vi "Send Create Arbitrary Sequence [SEQ].vi"(7 "Message Priority (Normal)":T1=enum."Normal", 8 "error in (no error)":errorcluster, 9 "waveform handles array (empty)":i32[](array[numeric]), 10 "loop counts array (empty)":i32[](array[numeric]), 11 "Message Enqueuer":refnum<class "Message Enqueuer.lvclass">) -> (0 "error out":errorcluster, 3 "Message Enqueuer out":refnum<class "Message Enqueuer.lvclass">)   [LabVIEW 2015, in "CS++Fgen.lvlib" / "Create Arbitrary Sequence [SEQ] Msg.lvclass"]
doc: "Sends the <B>CS++Fgen.lvlib:Create Arbitrary Sequence [SEQ] Msg.lvclass</B> message.\n\n<B>CS++Fgen.lvlib:CS++Fgen.lvclass:Create Arbitrary Sequence [SEQ].vi</B> Description:\n\nAn arbitrary sequence consists of multiple waveforms. For each waveform, you specify the number of times the function generator produces the waveform before proceeding to the next waveform. The number of times to repeat a specific waveform is called the loop count.\n \nThis VI creates an arbitrary sequence from an array of waveform handles and an array of corresponding loop counts. The VI returns a handle that identifies the sequence. You pass this handle to the IviFgen Configure Arbitrary Sequence [SEQ] VI to specify what arbitrary sequence you want the function generator to produce.\n\nNotes:\n\n(1) This VI is part of the IviFgenArbSeq [SEQ] extension group."
uses:
  Create Arbitrary Sequence [SEQ] Msg.lvclass
  <vilib>/ActorFramework/Message Enqueuer/Message Enqueuer.lvclass
  <vilib>/ActorFramework/Message Enqueuer/Message Priority.ctl
  Create Arbitrary Sequence [SEQ] Msg.lvclass/Create Arbitrary Sequence [SEQ] Msg.ctl
  <vilib>/ActorFramework/Message Enqueuer/Message Enqueuer.lvclass/Message Enqueuer.ctl
  <vilib>/ActorFramework/Message Priority Queue/Priority Enqueue.vi
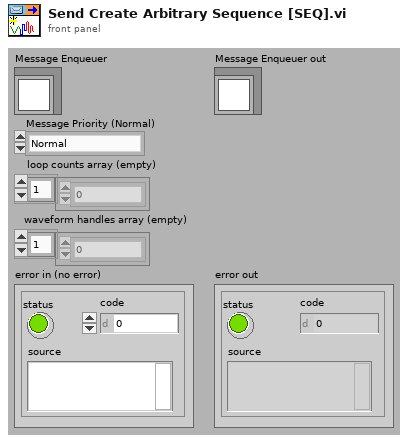
[diagram p1: front panel]
types:
  T1 = typedef "Actor Framework.lvlib/Message Enqueuer.lvclass/Message Priority.ctl" = enum16{"Low", "Normal", "High"}
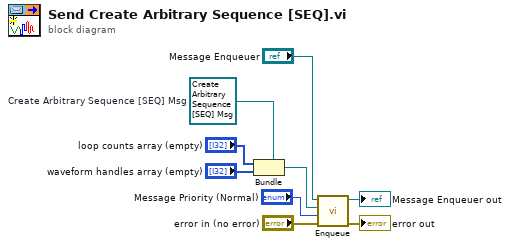
[diagram p0: block diagram]
diagram:
  w3 = refnum<class "Create Arbitrary Sequence [SEQ] Msg.lvclass"> refnum  # Create Arbitrary Sequence [SEQ] Msg
  n1 = Bundle(cluster=w3, "loop counts array (empty)", "waveform handles array (empty)") -> (w6:refnum<class "Create Arbitrary Sequence [SEQ] Msg.lvclass">)
  n2 = call <vilib>:"Enqueue.vi"("error in (no error)"="error in (no error)", "Message Priority (Normal)"="Message Priority (Normal)", "Message"=w6, "Message Enqueuer in"="Message Enqueuer") -> ("error out"=→"error out":errorcluster, "Message Enqueuer out"=→"Message Enqueuer out":refnum<class "Message Enqueuer.lvclass">)  [unwired: 6 in]
